vi "OverlayTextOnSavedImage.vi"(0 "Image":T2, 2 "Component Name":string, 9 "SNR/CNR Values":string, 11 "Error in (no error)":errorcluster) -> (4 "Image Dst Out":T2, 15 "Error out":errorcluster)   [LabVIEW 2021]
uses:
  <vilib>/vision/Image Controls.llb/IMAQ Image.ctl
panel:
  in  "Font, Size & Style":T1={"Desired Font (Application)"=enum."User-specified Font", "[User-specified Font]"={"Font Name"="Calibri", "Size"=48, "Strikeout?"=FALSE, "Italic?"=FALSE, "Underline?"=FALSE, "Outline?"=FALSE, "Shadow?"=TRUE, "Bold?"=FALSE, "Rotation Angle"=0.0}, "Horizontal Alignment"=0, "Vertical Alignment"=0} {"Horizontal Alignment" items=["Left", "Center", "Right"]; "Vertical Alignment" items=["Bottom", "Top", "Baseline"]}
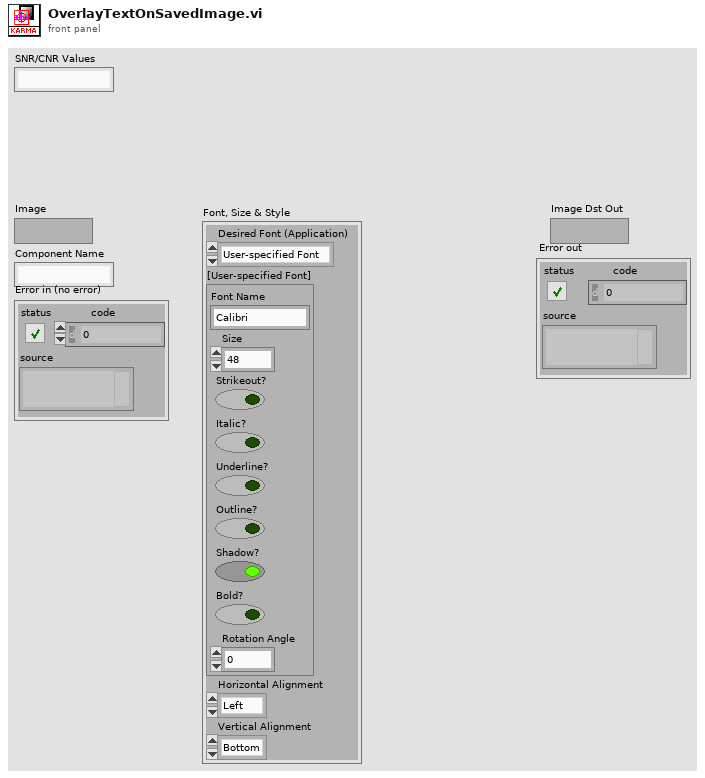
[diagram p1: front panel]
types:
  T1 = cluster{"Desired Font (Application)":enum16{"User-specified Font", "Application Font", "System Font", "Dialog Font"}, "[User-specified Font]":cluster{"Font Name":string, "Size":i16, "Strikeout?":bool, "Italic?":bool, "Underline?":bool, "Outline?":bool, "Shadow?":bool, "Bold?":bool, "Rotation Angle":dbl}, "Horizontal Alignment":i16, "Vertical Alignment":i16}
  T2 = typedef "IMAQ Image.ctl" = refnum<image>
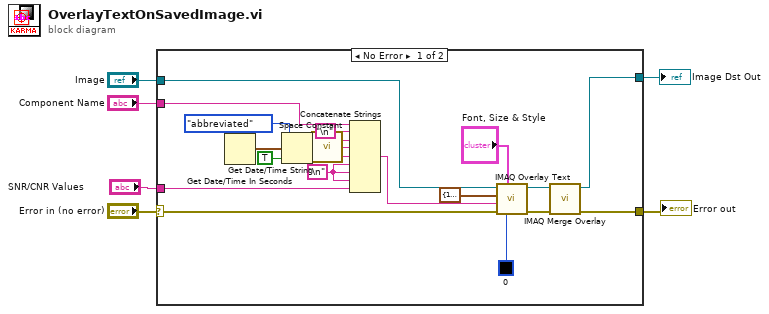
[diagram p0: block diagram]
diagram:
  n1 = case shown="No Error" "Error in (no error)" {
    selector: "Error in (no error)" -> [w9 w28]
    tunnel: "Image" -> [w13 w27]
    tunnel: [w12 w27] -> w5
    tunnel: "Component Name" -> [w11 _]
    tunnel: [w10 w28] -> w3
    tunnel: "SNR/CNR Values" -> [w8 _]
    frame No Error {
      w7 = "\n"
      n2 = Get Date/Time In Seconds() -> (seconds since 1Jan1904=w21:timestamp)
      n3 = Get Date/Time String(date format (0)=enum16{"short", "long", "abbreviated"}."abbreviated", seconds (now)=w21, want seconds? (F)=TRUE) -> (date string=w18:string, time string=w17:string)
      n4 = call <vilib>:"Space Constant.vi"() -> ("String"=w16:string)
      n5 = Concatenate Strings(w11, "\n", w18, w16, w17, w7, w7, w7, w8) -> (w14:string)
      n6 = call "IMAQ Overlay Text"("Text Color (black)"=u32 0, "Font, Size & Style"="Font, Size & Style", "error in (no error)"=w9, "String"=w14, "Origin"=cluster{"X":i32, "Y":i32} {"X"=100, "Y"=100}, "Image"=w13) -> ("error out"=w26:errorcluster, "Image Out"=w25:T2)  [unwired: 4 in]
      n7 = call "IMAQ Merge Overlay"("error in (no error)"=w26, "Image Src"=w25) -> ("error out"=w10:errorcluster, "Image Dst Out"=w12:T2)  [unwired: 8 in]
    }
    frame Error {
    }
  }
  "Image Dst Out" <- w5
  "Error out" <- w3
